vi "Regenerate gRPC code.vi"(11 "proto File Path":path) -> (0 "error out":errorcluster)   [LabVIEW 2021, in "Script gRPC.lvlib"]
uses:
  Script gRPC.lvlib
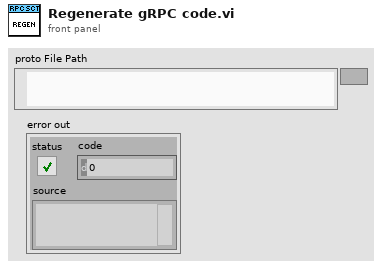
[diagram p1: front panel]
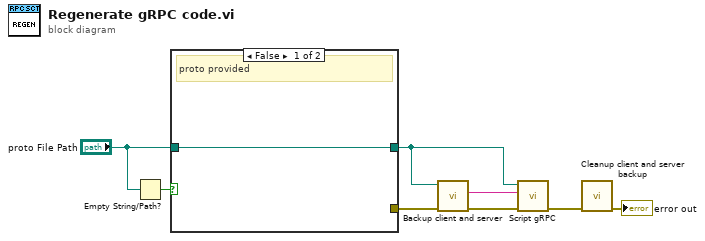
[diagram p0: block diagram]
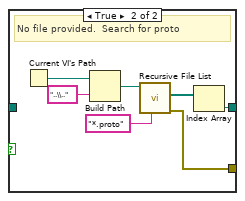
[diagram p2: hidden frame]
diagram:
  n1 = Empty String/Path?(string/path="proto File Path") -> (empty?=w1:bool)
  n2 = case shown="False" w1 {
    tunnel: [_ w12] -> w4
    tunnel: [w9 w10] -> w3
    tunnel: "proto File Path" -> [w9 _]
    frame False {
      # "proto provided"
    }
    frame True {
      # "No file provided.  Search for proto"
      n3 = Current VI's Path() -> (path=w15:path)
      n4 = Build Path(base path=w15, name or relative path="..\\.." ("String")) -> (appended path=w14:path)
      n5 = call <vilib>:"Recursive File List.vi"("pattern"="*.proto", "Folder Path"=w14) -> ("error out"=w12:errorcluster, "All Files in Dir"=w11:path[])  [unwired: 5 in, 3 out]
      n6 = Index Array(array=w11) -> (element=w10:path)  [unwired: 1 in]
    }
  }
  n7 = call "Backup client and server.vi"("error in"=w4, "proto File Path"=w3) -> ("error out"=w8:errorcluster, "Generated Library Name"=w7:string)  [unwired: 8 in]
  n8 = call "Script gRPC.vi"("error in"=w8, "Generated Library Name"=w7, "proto File Path"=w3) -> ("error out"=w6:errorcluster)  [unwired: 8 in]
  n9 = call "Cleanup client and server backup.vi"("error in"=w6) -> ("error out"=→"error out":errorcluster)  [unwired: 10 in]
